vi "WiFi lab coordinator Transparent v2.vi"() -> ()   [LabVIEW 2021]
uses:
  WiFi API Frame.ctl
  WiFi API Frame Type.ctl
  Protocol enum.ctl
  stop button.vi
  <vilib>/Utility/file.llb/Write Delimited Spreadsheet (string).vi
panel:
  in  "Response":string
  in  "stop":bool
  in  "Control string":string
  in  "Start session":bool
  in  "Destination port (hex)":u16=9750 step=1 format="%04x"
  in  "Source port (hex)":u16=2000 step=1 format="%04x"
  out "IPs":cluster{"Source IP":u8[], "RF Data":string}[](array[cluster])
  # "Session Configuration"
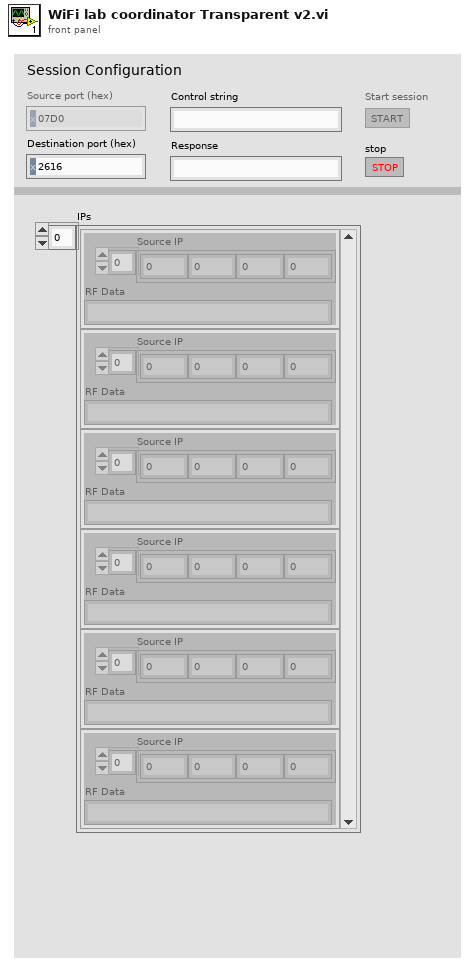
[diagram p1: front panel]
types:
  T1 = typedef "WiFi API Frame.ctl" = cluster{"Length":u16, "Frame Type":T2, "Payload":u8[], "Checksum":u8}
  T2 = typedef "WiFi API Frame Type.ctl" = u8
  T3 = enum8{"Enabled", "Disabled", "Disabled and Grayed Out"}
  T4 = typedef "Protocol enum.ctl" = enum8{"UDP", "TCP"}
  T5 = enum32{"invalid app kind", "Development System", "Run Time System", "Student Edition", "Embedded LabVIEW", "Evaluation", "Custom"}
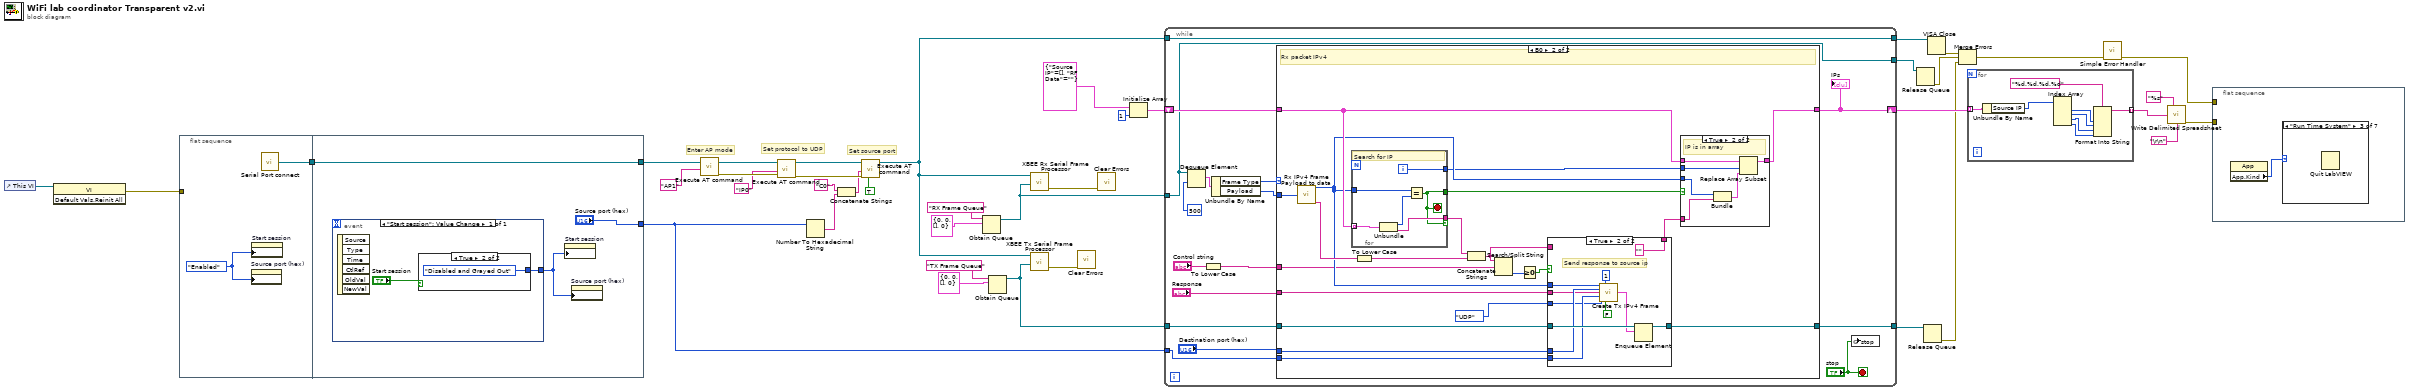
[diagram p0: block diagram]
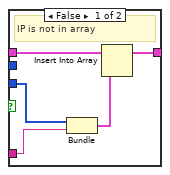
[diagram p10: hidden frame]
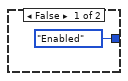
[diagram p11: hidden frame]
diagram:
  # "Set source port"
  # "Set protocol to UDP"
  # "Enter AP mode"
  n1 = control-ref of="This VI"() -> (w26:refnum<vi>)
  n2 = invoke class="VI" method="Default Vals.Reinit All"(reference=w26) -> (error out=w40:errorcluster)  [unwired: 2 in, 2 out]
  n3 = flat-sequence {
    tunnel: w40 -> [_]
    tunnel: [w41] -> w14
    tunnel: [w45] -> w27
    tunnel: w14 -> [w45]
    tunnel: ["Source port (hex)"] -> w1
    frame #0 {
      w42 = T3."Enabled" ("Disabled")
      n4 = property on="Source port (hex)" class="DigNum (strict)"("DisabledEnum"=w42) -> ()  [unwired: 2 in, 2 out]
      n5 = property on="Start session" class="Bool"("DisabledEnum"=w42) -> ()  [unwired: 2 in, 2 out]
      n6 = call "Serial Port connect.vi"() -> ("VISA resource out"=w41:refnum<visa-resource-name>)  [unwired: 1 in]
    }
    frame #1 {
      n7 = event shown="[0] \"Start session\": Value Change" {
        selector: _ -> [_]
        dyn-events: _ -> [_]
        timeout: _ -> [_]
        tunnel: [w47] -> w44
        event "Start session": Value Change {
          n8 = event-data() -> ()  [unwired: 1 in, 6 out]
          n9 = case shown="True" "Start session" {
            tunnel: [T3."Enabled" ("Disabled") T3."Disabled and Grayed Out" ("Disabled")] -> w47
            frame False {
            }
            frame True {
            }
          }
        }
      }
      n10 = property on="Start session" class="Bool"("DisabledEnum"=w44) -> ()  [unwired: 2 in, 2 out]
      n11 = property on="Source port (hex)" class="DigNum (strict)"("DisabledEnum"=w44) -> ()  [unwired: 2 in, 2 out]
    }
  }
  n12 = call "Execute AT command.vi"("AT Command"="AP1", "VISA resource in"=w27) -> ("error out"=w30:errorcluster, "VISA resource out"=w31:refnum<visa-resource-name>)  [unwired: 6 in, 1 out]
  n13 = call "Execute AT command.vi"("error in (no error)"=w30, "AT Command"="IP0", "VISA resource in"=w31) -> ("error out"=w24:errorcluster, "VISA resource out"=w25:refnum<visa-resource-name>)  [unwired: 5 in, 1 out]
  n14 = Number To Hexadecimal String(2:w1) -> (0:w20:string)  [unwired: 1 in]
  n15 = Concatenate Strings("C0" ("AT Command"), w20) -> (w21:string)
  n16 = call "Execute AT command.vi"("Exit AT mode"=TRUE, "error in (no error)"=w24, "AT Command"=w21, "VISA resource in"=w25) -> ("VISA resource out"=w23:refnum<visa-resource-name>)  [unwired: 4 in, 2 out]
  n17 = Obtain Queue(name (unnamed)="RX Frame Queue", element data type=T1 {"Length"=0, "Frame Type"=0, "Payload"=[], "Checksum"=0} ("API Frame")) -> (queue out=w35:refnum<queue>)  [unwired: 3 in, 2 out]
  n18 = Obtain Queue(name (unnamed)="TX Frame Queue", element data type=T1 {"Length"=0, "Frame Type"=0, "Payload"=[], "Checksum"=0} ("API Frame")) -> (queue out=w32:refnum<queue>)  [unwired: 3 in, 2 out]
  n19 = call "XBEE Rx Serial Frame Processor.vi"("RX Frame Queue"=w35, "VISA Serial Port"=w23) -> ("error out"=w11:errorcluster)  [unwired: 9 in]
  n20 = call "XBEE Tx Serial Frame Processor.vi"("TX Frame Queue"=w32, "VISA Serial Port"=w23) -> ("error out"=w10:errorcluster)  [unwired: 9 in]
  n21 = call <vilib>:"Clear Errors.vi"("error in (no error)"=w10) -> ()  [unwired: 5 in, 2 out]
  n22 = call <vilib>:"Clear Errors.vi"("error in (no error)"=w11) -> ()  [unwired: 5 in, 2 out]
  n23 = Initialize Array(cluster{"Source IP":u8[], "RF Data":string} {"Source IP"=[], "RF Data"=""}, 1 ("dimension size")) -> (w34:cluster{"Source IP":u8[], "RF Data":string}[])
  n24 = while {
    tunnel: w35 -> [w52]
    shift-right: [w54] -> w19
    shift-left: w34 -> [w62]
    tunnel: w32 -> [w61]
    tunnel: w23 -> [w60]
    tunnel: [w60] -> w9
    tunnel: [w52] -> w6
    tunnel: [w51] -> w7
    tunnel: w1 -> [w50]
    stop <- "stop" stop-if-true
    n25 = Dequeue Element(queue=w52, timeout in ms (-1)=500) -> (element=w65:T1)  [unwired: 1 in, 3 out]
    n26 = To Lower Case(string="Control string") -> (all lower case string=w57:string)
    n27 = Unbundle By Name(w65) -> ("Frame Type"=w64:T2, "Payload"=w63:u8[])
    n28 = case shown="B0" w64 {
      tunnel: w63 -> [_ w87]
      tunnel: w62 -> [w67 w85]
      tunnel: w57 -> [_ w74]
      tunnel: w61 -> [w66 w86]
      tunnel: "Destination port (hex)" -> [_ w84]
      tunnel: w50 -> [_ w83]
      tunnel: [w67 w82] -> w54
      tunnel: "Response" -> [_ w79]
      tunnel: [w66 w68] -> w51
      frame 0, Default {
      }
      frame 176 {
        # "Rx packet IPv4"
        n29 = call "Rx IPv4 Frame Payload to data.vi"("Payload array"=w87) -> ("Source IP"=w80:u8[], "RF data"=w81:string)  [unwired: 10 in, 3 out]
        n30 = for {
          tunnel: w80 -> [w114]
          tunnel: [w112] -> w78
          tunnel: w85 -> [w117] mode=indexing
          tunnel: [w116] -> w76
          tunnel: [w113] -> w77 if=w112
          i -> [w116]
          stop <- w112 stop-if-true
          # "Search for IP"
          n31 = Unbundle(w117) -> ("Source IP"=w115:u8[], "RF Data"=w113:string)
          n32 = Equal?(x=w114, y=w115) -> (x = y?=w112:bool)
        }
        n33 = To Lower Case(string=w81) -> (all lower case string=w75:string)
        n34 = Concatenate Strings(w77, w75) -> (w71:string)
        n35 = Search/Split String(string=w71, search string/char (-)=w74) -> (offset of match=w73:i32)  [unwired: 1 in, 2 out]
        n36 = Greater Or Equal To 0?(x=w73) -> (x >= 0?=w72:bool)
        n37 = case shown="True" w72 {
          tunnel: w86 -> [w88 w100]
          tunnel: w84 -> [_ w99]
          tunnel: w83 -> [_ w98]
          tunnel: w80 -> [_ w97]
          tunnel: Protocol_enum."UDP" ("Protocol") -> [_ w96]
          tunnel: w79 -> [_ w95]
          tunnel: w71 -> [w89 _]
          tunnel: [w89 ""] -> w70
          tunnel: [w88 w90] -> w68
          frame False {
          }
          frame True {
            # "Send response to source ip"
            n38 = call "Create Tx IPv4 Frame.vi"("Destination IP"=w97, "Frame ID"=u8 1, "Destination port"=w99, "RF data"=w95, "Source port"=w98, "Protocol"=w96, "Transmit options bitfield"=FALSE) -> ("TX IPv4 Frame"=w92:T1)  [unwired: 8 in]
            n39 = Enqueue Element(queue=w100, element=w92) -> (queue out=w90:refnum<queue>)  [unwired: 2 in, 2 out]
          }
        }
        n40 = case shown="True" w78 {
          tunnel: [w103 w111] -> w82
          tunnel: w85 -> [w105 w110]
          tunnel: w80 -> [w104 w109]
          tunnel: w70 -> [w101 w108]
          tunnel: w76 -> [_ w107]
          frame False {
            # "IP is not in array"
            n41 = Bundle("Source IP"=w104, w101) -> (w102:cluster{"Source IP":u8[], string})  [unwired: 1 in]
            n42 = Insert Into Array(array=w105, new element=w102) -> (w103:cluster{"Source IP":u8[], "RF Data":string}[])  [unwired: 1 in]
          }
          frame True {
            # "IP is in array"
            n43 = Bundle("Source IP"=w109, w108) -> (w106:cluster{"Source IP":u8[], string})  [unwired: 1 in]
            n44 = Replace Array Subset(array=w110, new element=w106, index=w107) -> (w111:cluster{"Source IP":u8[], "RF Data":string}[])
          }
        }
      }
    }
    "IPs" <- w54
    n45 = global write "stop button.vi" "stop"("stop") -> ()
  }
  n46 = Release Queue(queue=w6) -> (error out=w4:errorcluster)  [unwired: 2 in, 2 out]
  n47 = Release Queue(queue=w7) -> (error out=w3:errorcluster)  [unwired: 2 in, 2 out]
  n48 = VISA Close(VISA resource name=w9) -> (error out=w8:errorcluster)  [unwired: 1 in]
  n49 = Merge Errors(w8, w4, w3) -> (w5:errorcluster)
  n50 = for {
    tunnel: w19 -> [w125] mode=indexing
    tunnel: [w119] -> w17 mode=indexing
    n51 = Unbundle By Name(w125) -> ("Source IP"=w123:u8[])
    n52 = Index Array(array=w123) -> (element #1=w122:u8, element #2=w121:u8, element #3=w120:u8, element #4=w118:u8)  [unwired: 4 in]
    n53 = Format Into String(format string="%d.%d.%d.%d", w122, w121, w120, w118) -> (resulting string=w119:string)  [unwired: 2 in, 1 out]
  }
  n54 = call <vilib>:"Simple Error Handler.vi"("error in (no error)"=w5) -> ("error out"=w2:errorcluster)  [unwired: 4 in, 4 out]
  n55 = call-poly <vilib>:"Write Delimited Spreadsheet.vi"("format (%s)"="%s" ("format (%.3f)"), "1D data"=w17, "delimiter (\\t)"="\r\n") -> ("error out"=w15:errorcluster)  [unwired: 11 in, 1 out]
  n56 = flat-sequence {
    tunnel: w15 -> [_]
    tunnel: w2 -> [_]
    frame #0 {
      n57 = property class="App"() -> ("App.Kind"=w126:T5)  [unwired: 2 in, 2 out]
      n58 = case shown="\"Run Time System\"" w126 {
        frame "invalid app kind", Default {
        }
        frame "Development System" {
        }
        frame "Run Time System" {
          n59 = Quit LabVIEW() -> ()  [unwired: 1 in]
        }
        frame "Student Edition" {
        }
        frame "Embedded LabVIEW" {
        }
        frame "Evaluation" {
        }
        frame "Custom" {
        }
      }
    }
  }
